vi "Speed PI Control.vi"() -> ()   [LabVIEW 2011]
panel:
  in  "I-Gain":dbl(slide)=1.0 scale=0.0..2.0
  in  "P-Gain":dbl(slide)=1.0 scale=0.0..2.0
  in  "Setpoint Speed (rps)":dbl(slide) scale=-8.3..8.3
  out "Speed (rps)":dynamicdata(graph)
  in  "stop (F)":bool
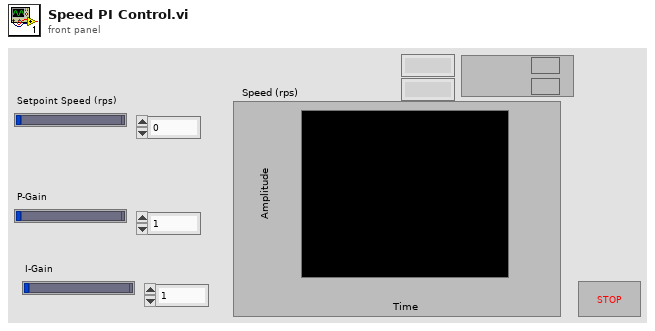
[diagram p1: front panel]
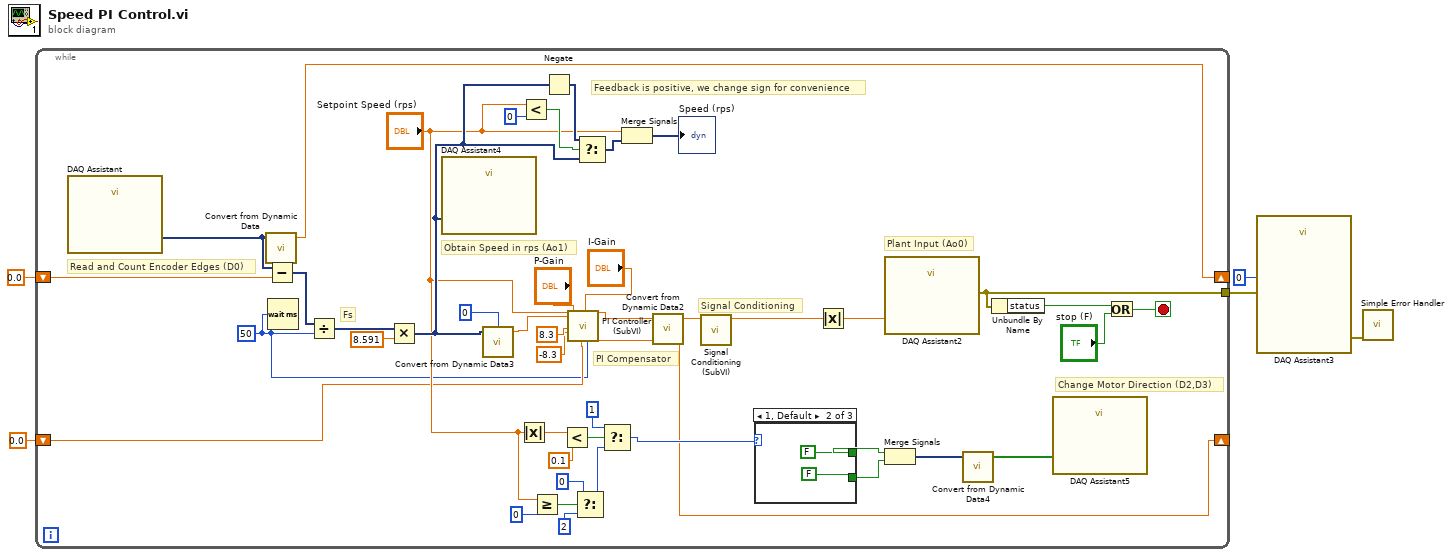
[diagram p0: block diagram]
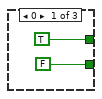
[diagram p2: hidden frame]
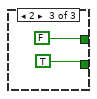
[diagram p3: hidden frame]
diagram:
  n1 = while {
    shift-right: [w49] -> _
    shift-left: 0.0 -> [w48]
    tunnel: [w44] -> w4
    shift-right: [w7] -> _
    shift-left: 0.0 -> [w8]
    stop <- w43 stop-if-true
    w6 = 50
    # "Feedback is positive, we change sign for convenience"
    # "Change Motor Direction (D2,D3)"
    # "Signal Conditioning"
    # "PI Compensator"
    # "Fs"
    # "Obtain Speed in rps (Ao1)"
    # "Read and Count Encoder Edges (D0)"
    # "Plant Input (Ao0)"
    n2 = call "DAQ Assistant"() -> ("data"=w40:dynamicdata)  [unwired: 16 in, 3 out]
    n3 = call "Convert from Dynamic Data"("Dynamic Data Type"=w40) -> ("Scalar"=w49:dbl)  [unwired: 3 in]
    n4 = Subtract(x=w40, y=w48) -> (x-y=w47:dynamicdata)
    n5 = Wait (ms)(milliseconds to wait=w6) -> ()  [unwired: 1 out]
    n6 = Divide(x=w47, y=w6) -> (x/y=w46:dynamicdata)
    n7 = Multiply(x=w46, y=8.591) -> (x*y=w17:dynamicdata)
    n8 = call "DAQ Assistant4"("data"=w17) -> ()  [unwired: 17 in, 2 out]
    n9 = call "Convert from Dynamic Data3"("Dynamic Data Type"=w17, "Channel"=0) -> ("Scalar"=w14:dbl)  [unwired: 2 in]
    n10 = Absolute Value(x="Setpoint Speed (rps)") -> (abs(x)=w30:dbl)
    n11 = Less?(x="Setpoint Speed (rps)", y=0) -> (x < y?=w18:bool)
    n12 = Greater Or Equal?(x="Setpoint Speed (rps)", y=0) -> (x >= y?=w33:bool)
    n13 = Negate(x=w17) -> (-x=w16:dynamicdata)
    n14 = Less?(x=w30, y=0.1) -> (x < y?=w28:bool)
    n15 = call "PI Controller (SubVI).vi"("sp"="Setpoint Speed (rps)", "pv"=w14, "maxim"=8.3, "minim"=-8.3, "p"="P-Gain", "errsum"=w8, "i"="I-Gain", "h"=w6) -> ("output variable"=w11:dbl, "errsum"=w7:dbl)  [unwired: 18 in]
    n16 = Select(t=0, s=w33, f=2) -> (s? t:f=w26:i32)
    n17 = Select(t=w16, s=w18, f=w17) -> (s? t:f=w19:dynamicdata)
    n18 = Select(t=1, s=w28, f=w26) -> (s? t:f=w23:i32)
    n19 = Merge Signals("Setpoint Speed (rps)", w19) -> (→"Speed (rps)":dynamicdata)
    n20 = call "Convert from Dynamic Data2"("Dynamic Data Type"=w11) -> ("Scalar"=w25:dbl)  [unwired: 3 in]
    n21 = call "Signal Conditioning (SubVI).vi"("Input"=w25) -> ("Output"=w22:dbl)  [unwired: 10 in]
    n22 = case shown="1, Default" w23 {
      tunnel: [TRUE FALSE FALSE] -> w36
      tunnel: [FALSE FALSE TRUE] -> w35
      frame 0 {
      }
      frame 1, Default {
      }
      frame 2 {
      }
    }
    n23 = Absolute Value(x=w22) -> (abs(x)=w24:dbl)
    n24 = call "DAQ Assistant2"("data"=w24) -> ("error out"=w44:errorcluster)  [unwired: 17 in, 1 out]
    n25 = Merge Signals(w36, w35) -> (w38:dynamicdata)
    n26 = call "Convert from Dynamic Data4"("Dynamic Data Type"=w38) -> ("Array"=w37:bool[])  [unwired: 3 in]
    n27 = Unbundle By Name(w44) -> ("status"=w41:bool)
    n28 = call "DAQ Assistant5"("data"=w37) -> ()  [unwired: 17 in, 2 out]
    n29 = Or(x=w41, y="stop (F)") -> (x .or. y?=w43:bool)
  }
  n30 = call "DAQ Assistant3"("data"=0, "error in"=w4) -> ("error out"=w2:errorcluster)  [unwired: 16 in, 1 out]
  n31 = call <vilib>:"Simple Error Handler.vi"("error in (no error)"=w2) -> ()  [unwired: 4 in, 5 out]
